vi "Teleop.vi"(10 "Match Info":T1={"Autonomous Elapsed Seconds"=0.0, "TeleOp Elapsed Seconds"=0.0, "Disabled Elapsed Seconds"=0.0, "Visited Autonomous"=FALSE, "Visited TeleOp"=FALSE, "Visited Disabled"=FALSE, "Autonomous Settings"={"Autonomous Style"=enum."Independent", "VI Refnum"=refnum}}, 11 "Call Context":T2) -> ()   [LabVIEW 2014]
doc: "This VI is called for each TeleOp packet received from the DS where the robot is not disabled. It is often used to read from the joysticks and update I/O or to update setpoints for timed control loops. It should complete and return within 20 milliseconds or it may miss DS packets."
uses:
  <vilib>/Rock Robotics/WPI/DriverStation/WPI_DriverStationDerivedRobotMode.ctl
  <vilib>/Rock Robotics/WPI/DriverStation/WPI_DriverStationMatch Info.ctl
  <vilib>/Rock Robotics/WPI/RobotDrive/WPI_RobotDriveGetSetRefNum.vi
  <vilib>/Rock Robotics/WPI/Joystick/WPI_JoystickGetSetRefNum.vi
  <vilib>/Rock Robotics/Network Tables/SD Write Numeric Array.vi
  <vilib>/Rock Robotics/Network Tables/SD Read Boolean.vi
  <vilib>/Rock Robotics/Network Tables/SD Read Number.vi
  <vilib>/Rock Robotics/Network Tables/SD Write Boolean Array.vi
panel:
  out "Sample Slider 0":dbl(slide) scale=0.0..5.0
  out "Sample Boolean 1":bool
  out "Sample Boolean 0":bool
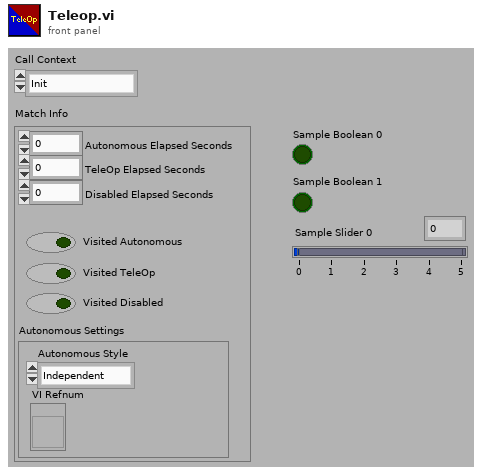
[diagram p1: front panel]
types:
  T1 = typedef "WPI_DriverStationMatch Info.ctl" = cluster{"Autonomous Elapsed Seconds":dbl, "TeleOp Elapsed Seconds":dbl, "Disabled Elapsed Seconds":dbl, "Visited Autonomous":bool, "Visited TeleOp":bool, "Visited Disabled":bool, "Autonomous Settings":cluster{"Autonomous Style":enum16{"Iterative", "Independent"}, "VI Refnum":refnum<vi>}}
  T2 = typedef "WPI_DriverStationDerivedRobotMode.ctl" = enum16{"Init", "Execute", "Stop"}
  T3 = typedef "WPI_JoystickDevRef.ctl" = cluster{"Device":T4}
  T4 = typedef "WPI_JoystickDeviceEnum.ctl" = enum16{"USB 0", "USB 1", "USB 2", "USB 3", "USB 4", "USB 5"}
  T5 = typedef "WPI_RobotDriveDevRef.ctl" = cluster{"DevStatus":errorcluster, "Motors[]":T6[], "Square Inputs":bool, "Max Output":dbl}
  T6 = typedef "WPI_MotorControlDeviceRef.ctl" = cluster{"DeviceStatus":errorcluster, "Type":T7, "PWM":cluster{"Controller":T8, "PWM Channel":T9, "DeadBand":T10}, "CAN":cluster{"Device Number":u8, "Control Mode":T11, "Semaphore":T12, "Max Vout":dbl, "TalonSRX Control Mode":T13}, "Invert":bool, "TransformRef":T14, "InvTransformRef":T14}
  T7 = typedef "WPI_MotorControlType.ctl" = enum16{"PWM", "CAN", "CANTalonSRX"}
  T8 = typedef "FPGA_TypedefDigitalModule.ctl" = enum16{"Controller 1"}
  T9 = typedef "FPGA_DIOPWMChannel.ctl" = enum8{"PWM 0", "PWM 1", "PWM 2", "PWM 3", "PWM 4", "PWM 5", "PWM 6", "PWM 7", "PWM 8", "PWM 9", "PWM MXP 0", "PWM MXP 1", "PWM MXP 2", "PWM MXP 3", "PWM MXP 4", "PWM MXP 5", "PWM MXP 6", "PWM MXP 7", "PWM MXP 8", "PWM MXP 9", "Invalid"}
  T10 = typedef "WPI_PWMDeadband.ctl" = cluster{"Name":string, "maxPositivePwm":i32, "minPositivePwm":i32, "centerPwm":i32, "maxNegativePwm":i32, "minNegativePwm":i32, "angularRange":u16}
  T11 = typedef "WPI_CANJaguar_ControlMode.ctl" = enum8{"Percent VBus", "Current", "Speed", "Position", "Voltage"}
  T12 = typedef "Semaphore RefNum" = refnum<k1>
  T13 = typedef "WPI_CANTalonSRX_APIControlMode.ctl" = enum8{"Percent VBus", "Speed", "Position", "Slave", "Unchanged / Invalid"}
  T14 = typedef "WPI_PWMTransform_ConPane.ctl" = refnum<vi>
  T15 = cluster{"Button 1":bool, "Button 2":bool, "Button 3":bool, "Button 4":bool, "Button 5":bool, "Button 6":bool, "Button 7":bool, "Button 8":bool, "Button 9":bool, "Button 10":bool, "Button 11":bool, "Button 12":bool}
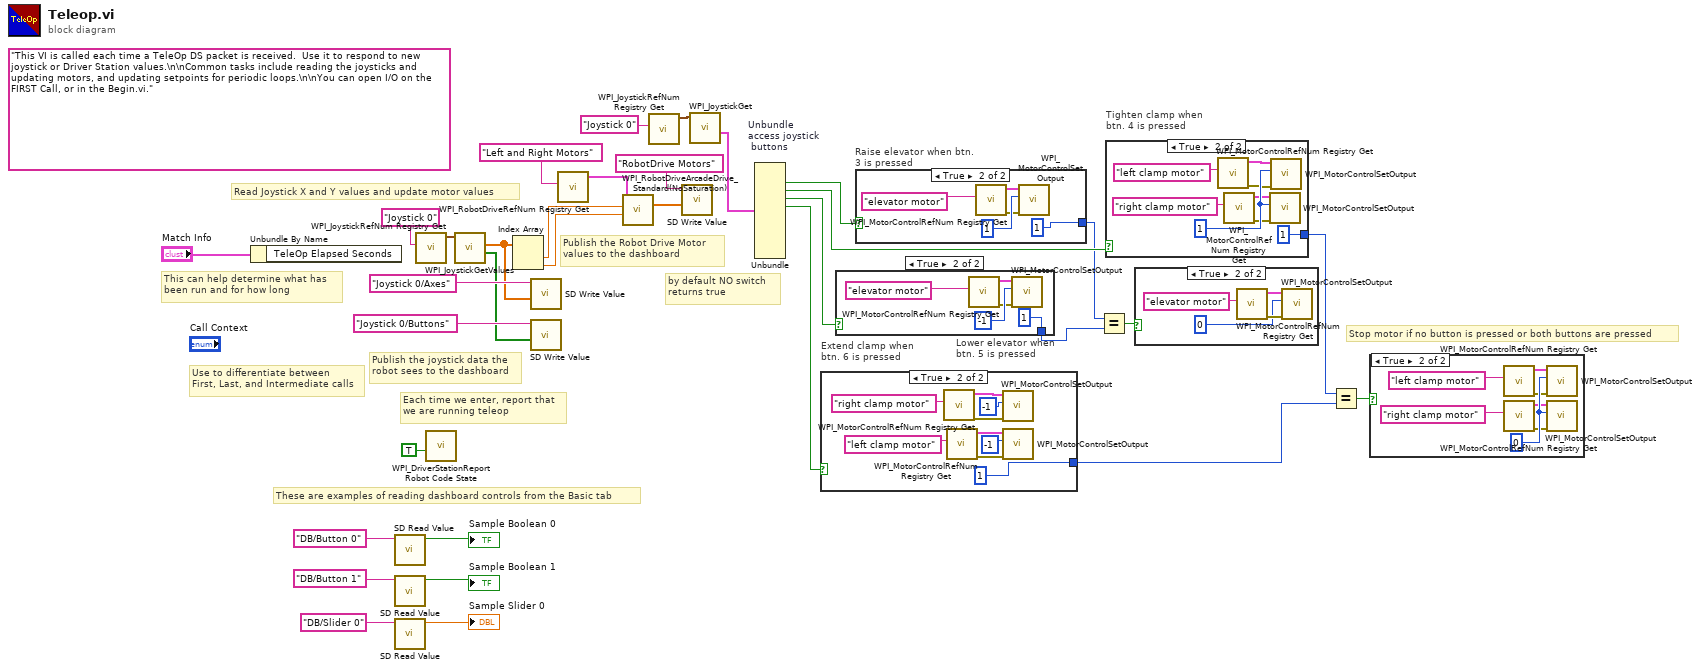
[diagram p0: block diagram]
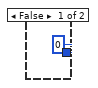
[diagram p4: hidden frame]
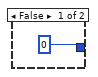
[diagram p5: hidden frame]
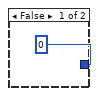
[diagram p6: hidden frame]
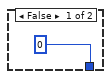
[diagram p7: hidden frame]
diagram:
  (unwired) "This VI is called each time a TeleOp DS packet is received.  Use it to respond to new joystick or Driver Station values.\n\nCommon tasks include reading the joysticks and updating motors, and updating setpoints for periodic loops.\n\nYou can open I/O on the FIRST Call, or in the Begin.vi."
  # "Stop motor if no button is pressed or both buttons are pressed"
  # "by default NO switch\nreturns true"
  # "These are examples of reading dashboard controls from the Basic tab"
  # "Publish the Robot Drive Motor\nvalues to the dashboard"
  # "Publish the joystick data the\nrobot sees to the dashboard"
  # "Each time we enter, report that\nwe are running teleop"
  # "Use to differentiate between\nFirst, Last, and Intermediate calls"
  # "This can help determine what has\nbeen run and for how long"
  # "Read Joystick X and Y values and update motor values"
  n1 = Unbundle By Name("Match Info") -> ()  [unwired: 1 out]
  n2 = call-poly <vilib>:"SD Read Value.vi"("Name"="DB/Button 0" ("refnum name")) -> ("Boolean"=→"Sample Boolean 0":bool)  [unwired: 8 in, 2 out]
  n3 = call-poly <vilib>:"SD Read Value.vi"("Name"="DB/Button 1" ("refnum name")) -> ("Boolean"=→"Sample Boolean 1":bool)  [unwired: 8 in, 2 out]
  n4 = call-poly <vilib>:"SD Read Value.vi"("Name"="DB/Slider 0" ("refnum name")) -> ("Numeric"=→"Sample Slider 0":dbl)  [unwired: 8 in, 2 out]
  n5 = call <vilib>:"WPI_JoystickRefNum Registry Get.vi"("refnum name"="Joystick 0") -> ("JoystickDevRef"=w29:T3)  [unwired: 1 in, 9 out]
  n6 = call <vilib>:"WPI_DriverStationReport Robot Code State.vi"("TeleOp"=TRUE ("Autonomous")) -> ()  [unwired: 10 in, 1 out]
  n7 = call <vilib>:"WPI_JoystickGetValues.vi"("JoystickDevRef"=w29) -> ("Buttons"=w15:bool[], "Axes"=w17:dbl[])  [unwired: 6 in, 3 out]
  n8 = Index Array(array=w17) -> (element #1=w9:dbl, element #2=w20:dbl)  [unwired: 2 in]
  n9 = call-poly <vilib>:"SD Write Value.vi"("Numeric Array"=w17, "Name"="Joystick 0/Axes") -> ()  [unwired: 8 in, 2 out]
  n10 = call-poly <vilib>:"SD Write Value.vi"("Boolean Array"=w15, "Name"="Joystick 0/Buttons") -> ()  [unwired: 8 in, 2 out]
  n11 = call <vilib>:"WPI_RobotDriveRefNum Registry Get.vi"("refnum name"="Left and Right Motors") -> ("RobotDriveDevRef"=w31:T5)  [unwired: 1 in, 9 out]
  n12 = call <vilib>:"WPI_RobotDriveArcadeDrive_Standard(NoSaturation).vi"("Y axis value"=w20, "X axis value"=w9, "RobotDriveDevRef"=w31) -> ("Motor Values"=w19:dbl[])  [unwired: 1 in, 7 out]
  n13 = call <vilib>:"WPI_JoystickRefNum Registry Get.vi"("refnum name"="Joystick 0") -> ("JoystickDevRef"=w14:T3)  [unwired: 9 in, 1 out]
  n14 = call-poly <vilib>:"SD Write Value.vi"("Numeric Array"=w19, "Name"="RobotDrive Motors") -> ()  [unwired: 8 in, 2 out]
  n15 = call <vilib>:"WPI_JoystickGet.vi"("JoystickDevRef"=w14) -> ("Buttons"=w10:T15)  [unwired: 1 in, 5 out]
  n16 = Unbundle "Unbundle\naccess joystick\n buttons"(w10) -> ("Button 3"=w2:bool, "Button 4"=w13:bool, "Button 5"=w1:bool, "Button 6"=w12:bool)  [unwired: 8 out]
  n17 = case "Extend clamp when \nbtn. 6 is pressed" shown="True" w12 {
    tunnel: [0 1] -> w4
    frame False {
    }
    frame True {
      n18 = call <vilib>:"WPI_MotorControlRefNum Registry Get.vi"("refnum name"="right clamp motor") -> ("error out"=w37:errorcluster, "MotorControlDevRef"=w36:T6)  [unwired: 9 in]
      n19 = call <vilib>:"WPI_MotorControlRefNum Registry Get.vi"("refnum name"="left clamp motor") -> ("error out"=w41:errorcluster, "MotorControlDevRef"=w40:T6)  [unwired: 9 in]
      n20 = call <vilib>:"WPI_MotorControlSetOutput.vi"("error in (no error)"=w37, "Output"=-1, "MotorControlDevRef"=w36) -> ()  [unwired: 6 in, 3 out]
      n21 = call <vilib>:"WPI_MotorControlSetOutput.vi"("error in (no error)"=w41, "Output"=-1, "MotorControlDevRef"=w40) -> ()  [unwired: 6 in, 3 out]
    }
  }
  n22 = case "Lower elevator when btn. 5 is pressed" shown="True" w1 {
    tunnel: [0 1] -> w8
    frame False {
    }
    frame True {
      n23 = call <vilib>:"WPI_MotorControlRefNum Registry Get.vi"("refnum name"="elevator motor") -> ("error out"=w48:errorcluster, "MotorControlDevRef"=w47:T6)  [unwired: 9 in]
      n24 = call <vilib>:"WPI_MotorControlSetOutput.vi"("error in (no error)"=w48, "Output"=-1, "MotorControlDevRef"=w47) -> ()  [unwired: 6 in, 3 out]
    }
  }
  n25 = case "Raise elevator when btn. 3 is pressed" shown="True" w2 {
    tunnel: [0 1] -> w7
    frame False {
    }
    frame True {
      n26 = call <vilib>:"WPI_MotorControlRefNum Registry Get.vi"("refnum name"="elevator motor") -> ("error out"=w54:errorcluster, "MotorControlDevRef"=w52:T6)  [unwired: 9 in]
      n27 = call <vilib>:"WPI_MotorControlSetOutput.vi"("error in (no error)"=w54, "Output"=1, "MotorControlDevRef"=w52) -> ()  [unwired: 6 in, 3 out]
    }
  }
  n28 = Equal?(x=w7, y=w8) -> (x = y?=w6:bool)
  n29 = case "Tighten clamp when \nbtn. 4 is pressed" shown="True" w13 {
    tunnel: [0 1] -> w5
    frame False {
    }
    frame True {
      w64 = 1
      n30 = call <vilib>:"WPI_MotorControlRefNum Registry Get.vi"("refnum name"="left clamp motor") -> ("error out"=w63:errorcluster, "MotorControlDevRef"=w62:T6)  [unwired: 9 in]
      n31 = call <vilib>:"WPI_MotorControlRefNum Registry Get.vi"("refnum name"="right clamp motor") -> ("error out"=w60:errorcluster, "MotorControlDevRef"=w59:T6)  [unwired: 9 in]
      n32 = call <vilib>:"WPI_MotorControlSetOutput.vi"("error in (no error)"=w60, "Output"=w64, "MotorControlDevRef"=w59) -> ()  [unwired: 6 in, 3 out]
      n33 = call <vilib>:"WPI_MotorControlSetOutput.vi"("error in (no error)"=w63, "Output"=w64, "MotorControlDevRef"=w62) -> ()  [unwired: 6 in, 3 out]
    }
  }
  n34 = case shown="True" w6 {
    frame False {
    }
    frame True {
      n35 = call <vilib>:"WPI_MotorControlRefNum Registry Get.vi"("refnum name"="elevator motor") -> ("error out"=w68:errorcluster, "MotorControlDevRef"=w67:T6)  [unwired: 9 in]
      n36 = call <vilib>:"WPI_MotorControlSetOutput.vi"("error in (no error)"=w68, "Output"=0, "MotorControlDevRef"=w67) -> ()  [unwired: 6 in, 3 out]
    }
  }
  n37 = Equal?(x=w5, y=w4) -> (x = y?=w3:bool)
  n38 = case shown="True" w3 {
    frame False {
    }
    frame True {
      w75 = 0
      n39 = call <vilib>:"WPI_MotorControlRefNum Registry Get.vi"("refnum name"="left clamp motor") -> ("error out"=w74:errorcluster, "MotorControlDevRef"=w73:T6)  [unwired: 9 in]
      n40 = call <vilib>:"WPI_MotorControlRefNum Registry Get.vi"("refnum name"="right clamp motor") -> ("error out"=w71:errorcluster, "MotorControlDevRef"=w70:T6)  [unwired: 9 in]
      n41 = call <vilib>:"WPI_MotorControlSetOutput.vi"("error in (no error)"=w74, "Output"=w75, "MotorControlDevRef"=w73) -> ()  [unwired: 6 in, 3 out]
      n42 = call <vilib>:"WPI_MotorControlSetOutput.vi"("error in (no error)"=w71, "Output"=w75, "MotorControlDevRef"=w70) -> ()  [unwired: 6 in, 3 out]
    }
  }
